vi "0to10.vi"(11 "Numeric":i32) -> (3 "Boolean":bool)   [LabVIEW 2014]
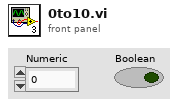
[diagram p1: front panel]
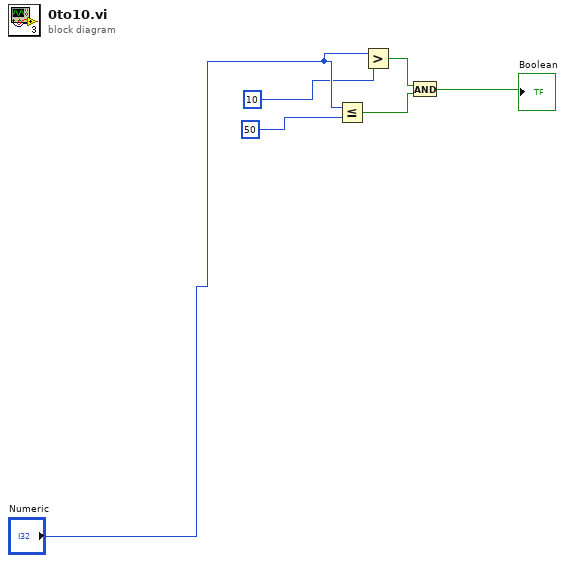
[diagram p0: block diagram]
diagram:
  n1 = Less Or Equal?(x="Numeric", y=50) -> (x <= y?=w1:bool)
  n2 = Greater?(x="Numeric", y=10) -> (0:w2:bool)
  n3 = And(x=w2, y=w1) -> (x .and. y?=→"Boolean":bool)
